vi "Compute LUT.vi"(11 "Hub Distance (ft)":dbl) -> (2 "Hood Setpoint":dbl, 3 "Shooter RPM":dbl)   [LabVIEW 2025]
uses:
  Get Shooter LUT.vi
  Get Hood LUT.vi
  Get Distance LUT.vi
  <vilib>/Analysis/NI_AALPro.lvlib
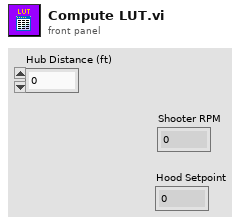
[diagram p1: front panel]
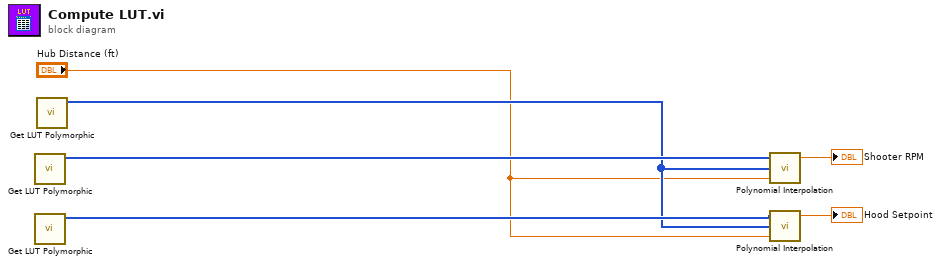
[diagram p0: block diagram]
diagram:
  n1 = call-poly "Get LUT Polymorphic.vi"() -> ("LUT Out"=w6:i32[])  [unwired: 10 in, 1 out]
  n2 = call-poly "Get LUT Polymorphic.vi"() -> ("LUT Out"=w4:i32[])  [unwired: 10 in, 1 out]
  n3 = call-poly "Get LUT Polymorphic.vi"() -> ("LUT Out"=w3:i32[])  [unwired: 10 in, 1 out]
  n4 = call <vilib>:"Polynomial Interpolation.vi"("x value"="Hub Distance (ft)", "X"=w3, "Y"=w6) -> ("interpolation value"=→"Shooter RPM":dbl)  [unwired: 2 out]
  n5 = call <vilib>:"Polynomial Interpolation.vi"("x value"="Hub Distance (ft)", "X"=w3, "Y"=w4) -> ("interpolation value"=→"Hood Setpoint":dbl)  [unwired: 2 out]
